vi "ClassPanel.vi"(8 "error in (no error)":errorcluster caption="entrée d'erreur (pas d'erreur)", 11 "Monospec50.lvclass":refnum<class "Monospec50.lvclass">) -> (0 "error out":errorcluster caption="sortie d'erreur", 3 "Monospec50.lvclass Out":refnum<class "Monospec50.lvclass">)   [LabVIEW 2012, in "Monospec50.lvclass"]
uses:
  Monospec50.lvclass
  BaseDevice/Accessor/GetClassEvent.vi
panel:
  in  "Annuler":bool caption="MiseAJour"
  out "PosAct":dbl caption="Position\nActuelle (nm)"
  out "Moving":bool caption="Déplacement\nen cours"
  in  "PosDem":dbl=300.0 caption="Position (nm)" min=300.0 max=730.0 step=0.01
  in  "Stop":bool
  in  "MiseAJour":bool
  out "Init Program":bool
  # "Monospec 50"
  # "this MUST labeled with class name"
  # "this MUST be present and labeled \"Stop\""
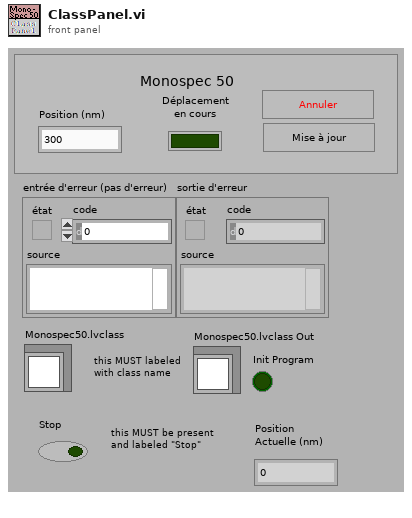
[diagram p1: front panel]
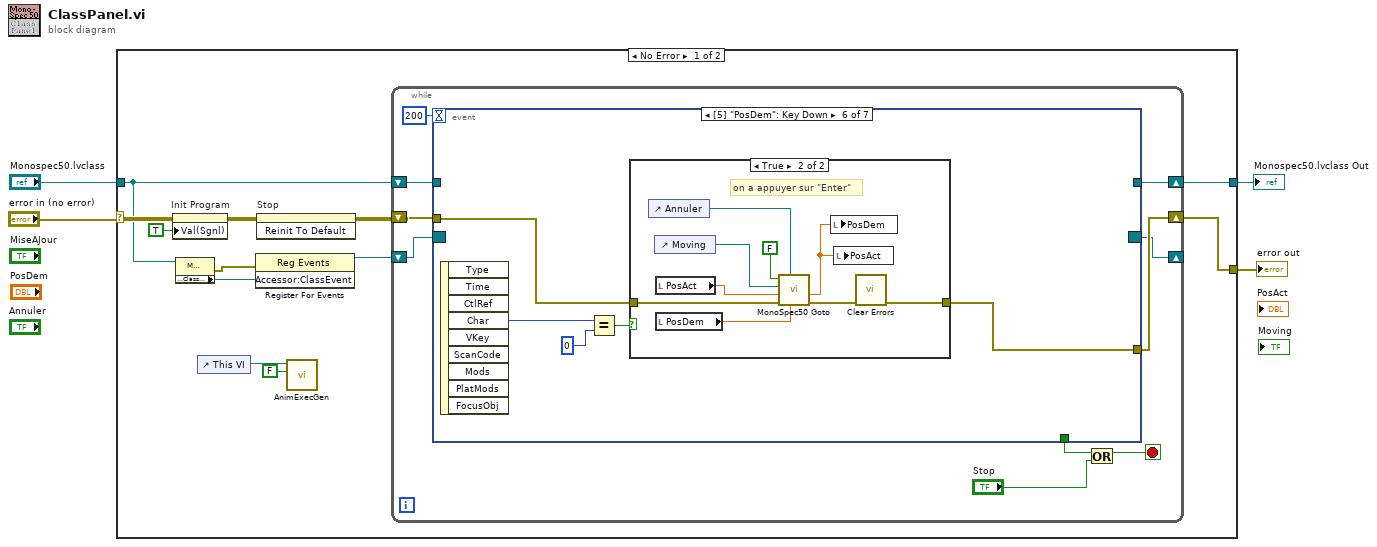
[diagram p0: block diagram]
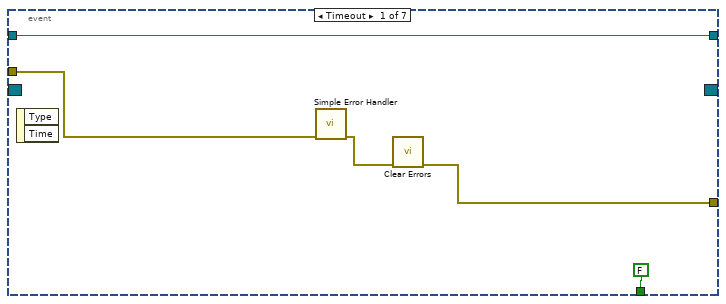
[diagram p2: hidden frame]
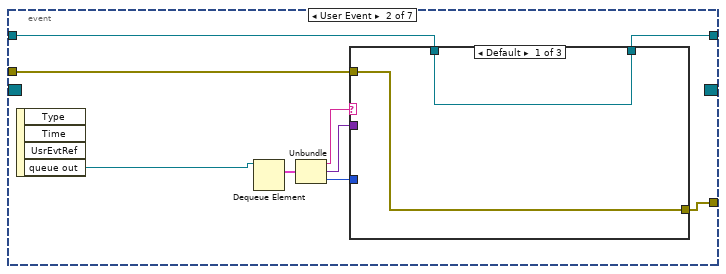
[diagram p3: hidden frame]
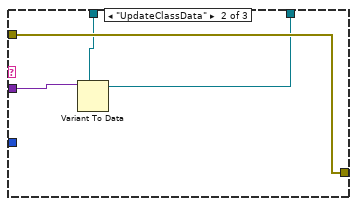
[diagram p4: hidden frame]
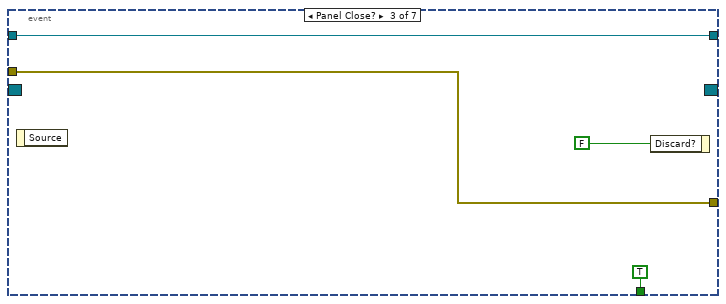
[diagram p6: hidden frame]
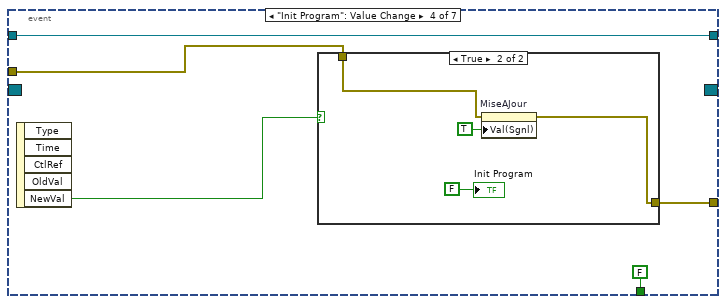
[diagram p7: hidden frame]
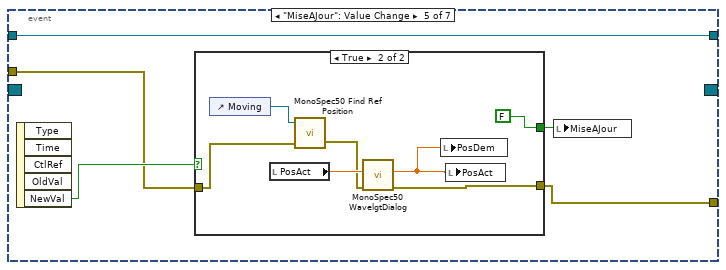
[diagram p9: hidden frame]
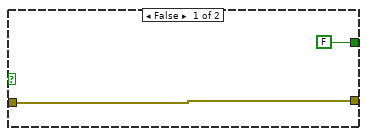
[diagram p10: hidden frame]
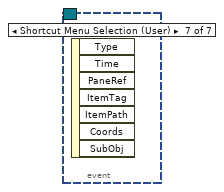
[diagram p12: hidden frame]
diagram:
  n1 = case shown="No Error" "error in (no error)" {
    selector: "error in (no error)" -> [w13 w93]
    tunnel: [w16 w93] -> w3
    tunnel: "Monospec50.lvclass" -> [w8 w92]
    tunnel: [w14 w92] -> w1
    frame No Error {
      n2 = property on="Init Program" class="Bool (strict)"(error in=w13, "Val(Sgnl)"=TRUE ("Valeur (Signalisation)")) -> (error out=w12:errorcluster)  [unwired: 1 in, 1 out]
      n3 = property class="Monospec50.lvclass"(reference=w8) -> (error out=w10:errorcluster, "Accessor:ClassEvent"=w9:refnum<user-event>)  [unwired: 1 in, 1 out]
      n4 = control-ref of="This VI"() -> (w5:refnum<vi>)
      n5 = register-events(error in=w10, w9) -> (reference out=w7:refnum<event-registration>)  [unwired: 1 in, 1 out]
      n6 = invoke on="Stop" class="Bool (strict)" method="Reinit To Default"(error in=w12) -> (error out=w11:errorcluster)  [unwired: 2 in, 2 out]
      n7 = call <userlib>:"AnimExecGen.vi"("Animer l'exécution ?"=FALSE, "ViRef"=w5) -> ()  [unwired: 9 in, 1 out]
      n8 = while {
        shift-right: [w24] -> w16
        shift-left: w11 -> [w25]
        shift-right: [w21] -> w14
        shift-left: w8 -> [w23]
        shift-right: [w17] -> _
        shift-left: w7 -> [w18]
        stop <- w20 stop-if-true
        n9 = event shown="[5] \"PosDem\": Key Down" {
          selector: w18 -> [_ _ _ _ _ _ _]
          dyn-events: [_ _ _ _ _ _ _] -> w17
          timeout: 200 -> [_ _ _ _ _ _ _]
          tunnel: w25 -> [w29 w39 w50 w56 w63 w79 _]
          tunnel: [w27 w33 w50 w55 w65 w77 _] -> w24
          tunnel: w23 -> [w30 w40 w49 w54 w67 _ _]
          tunnel: [FALSE _ TRUE FALSE _ _ _] -> w22
          tunnel: [w30 w32 w49 w54 w67 _ _] -> w21
          event Timeout {
            n10 = event-data() -> ()  [unwired: 1 in, 2 out]
            n11 = call <vilib>:"Simple Error Handler.vi"("error in (no error)"=w29) -> ("error out"=w28:errorcluster)  [unwired: 4 in, 4 out]
            n12 = call <vilib>:"Clear Errors.vi"("error in (no error)"=w28) -> ("error out"=w27:errorcluster)  [unwired: 6 in]
          }
          event User Event {
            n13 = event-data() -> ("queue out"=w37:refnum<queue>)  [unwired: 1 in, 3 out]
            n14 = Dequeue Element(queue=w37) -> (element=w38:cluster{"Message":string, "Data":variant, i32})  [unwired: 2 in, 3 out]
            n15 = Unbundle(w38) -> ("Message"=w36:string, "Data"=w35:variant, w34:i32)
            n16 = case shown="Default" w36 {
              tunnel: w39 -> [w42 w46 w47]
              tunnel: w35 -> [_ w45 _]
              tunnel: w40 -> [w41 w44 w48]
              tunnel: [w41 w43 w48] -> w32
              tunnel: [w42 w46 w47] -> w33
              tunnel: w34 -> [_ _ _]
              frame Default {
              }
              frame "UpdateClassData" {
                n17 = Variant To Data(type=w44, Variant=w45) -> (data=w43:refnum<class "Monospec50.lvclass">)  [unwired: 1 in, 1 out]
              }
              frame "MeasDone" {
              }
            }
          }
          event Panel Close? {
            n18 = event-data() -> ()  [unwired: 1 in, 1 out]
            n19 = event-data("Discard?"=FALSE ("Rejeter ?")) -> ()  [unwired: 1 in, 1 out]
          }
          event "Init Program": Value Change {
            n20 = event-data() -> ("NewVal"=w57:bool)  [unwired: 1 in, 4 out]
            n21 = case shown="True" w57 {
              tunnel: w56 -> [w58 w60]
              tunnel: [w58 w59] -> w55
              frame False {
              }
              frame True {
                n22 = property on="MiseAJour" class="Bool (strict)"(error in=w60, "Val(Sgnl)"=TRUE ("Value (Signaling)")) -> (error out=w59:errorcluster)  [unwired: 1 in, 1 out]
                "Init Program" <- FALSE
              }
            }
          }
          event "MiseAJour": Value Change {
            n23 = event-data() -> ("NewVal"=w64:bool)  [unwired: 1 in, 4 out]
            n24 = case shown="True" w64 {
              tunnel: w63 -> [w69 w72]
              tunnel: [w69 w76] -> w65
              tunnel: [FALSE FALSE] -> w66
              frame False {
              }
              frame True {
                n25 = control-ref of="Moving"() -> (w70:refnum<vi>)
                n26 = local read "PosAct"() -> (w75:dbl)
                n27 = call <userlib>:"MonoSpec50 Find Ref Position.vi"("error in"=w72, "Moving Ref"=w70) -> ("error out"=w71:errorcluster)  [unwired: 1 in, 1 out]
                n28 = call <userlib>:"MonoSpec50 WavelgtDialog.vi"("error in (no error)"=w71, "PosAct"=w75) -> ("error out"=w76:errorcluster, "PosAct Out"=w73:dbl)  [unwired: 4 in]
                n29 = local write "PosDem"(w73) -> ()
                n30 = local write "PosAct"(w73) -> ()
              }
            }
            n31 = local write "MiseAJour"(w66) -> ()
          }
          event "PosDem": Key Down {
            n32 = event-data() -> ("Char"=w78:i16)  [unwired: 1 in, 8 out]
            n33 = Equal?(x=w78, y=i16 0) -> (x = y?=w80:bool)
            n34 = case shown="True" w80 {
              tunnel: [w82 w88] -> w77
              tunnel: w79 -> [w82 w91]
              frame False {
              }
              frame True {
                # "on a appuyer sur \"Enter\""
                n35 = control-ref of="Annuler"() -> (w83:refnum<vi>)
                n36 = control-ref of="Moving"() -> (w87:refnum<vi>)
                n37 = local read "PosAct"() -> (w90:dbl)
                n38 = local read "PosDem"() -> (w86:dbl)
                n39 = call <userlib>:"MonoSpec50 Goto.vi"("PosDem"=w86, "Abort Ref"=w83, "error in (no error)"=w91, "PosAct"=w90, "Moving Ref"=w87, "Ask Act Pos"=FALSE) -> ("error out"=w89:errorcluster, "PosAct Out"=w84:dbl)  [unwired: 2 in]
                n40 = local write "PosDem"(w84) -> ()
                n41 = local write "PosAct"(w84) -> ()
                n42 = call <vilib>:"Clear Errors.vi"("error in (no error)"=w89) -> ("error out"=w88:errorcluster)  [unwired: 6 in]
              }
            }
          }
          event Shortcut Menu Selection (User) {
            n43 = event-data() -> ()  [unwired: 1 in, 7 out]
          }
        }
        n44 = Or(x=w22, y="Stop") -> (x .or. y?=w20:bool)
      }
    }
    frame Error {
    }
  }
  "error out" <- w3
  "Monospec50.lvclass Out" <- w1
